vi "Start BaseActor.vi"() -> ()   [LabVIEW 2013, in "CS++Core-Examples.lvlib"]
doc: "This example illustrates how to start an actor via Factory and to send an Stop-Message on stop."
uses:
  CS++Core-Examples.lvlib
  Core/Classes/CS++BaseClasses/Factory/CS++Factory.lvclass
  Core/Classes/CS++BaseClasses/Factory/CS++Factory.lvclass/CS++Factory.ctl
  <vilib>/ActorFramework/Message Queue/Message Queue.lvclass/Message Queue.ctl
  <vilib>/ActorFramework/Message Enqueuer/Message Enqueuer.lvclass/Message Enqueuer.ctl
  <vilib>/ActorFramework/Message Enqueuer/Enqueue.vi
  <vilib>/Utility/config.llb/Read Key (String).vi
  <vilib>/ActorFramework/Message Priority Queue/Priority Enqueue.vi
  <vilib>/ActorFramework/Stop Msg/Stop Msg.lvclass
  <vilib>/ActorFramework/Actor/Actor.lvclass
  <vilib>/ActorFramework/Message Queue/Message Queue.lvclass
  Core/Libraries/MessageLogger/CS++MessageLogger.lvlib
  <vilib>/Utility/config.llb/NI_LVConfig.lvlib
panel:
  in  "Configuration File":path=path "C:/User/Brand/Git/CSPP/Core/CS++Example.ini"
  in  "Stop Button":bool
  in  "Object Name":string="myActor_0"
  out "Attributes found?":bool
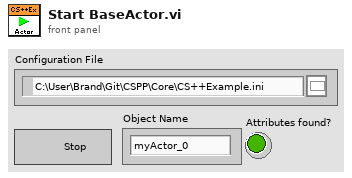
[diagram p1: front panel]
types:
  T1 = typedef "NI_LVConfig.lvlib/Config Data RefNum.ctl" = refnum<k1>
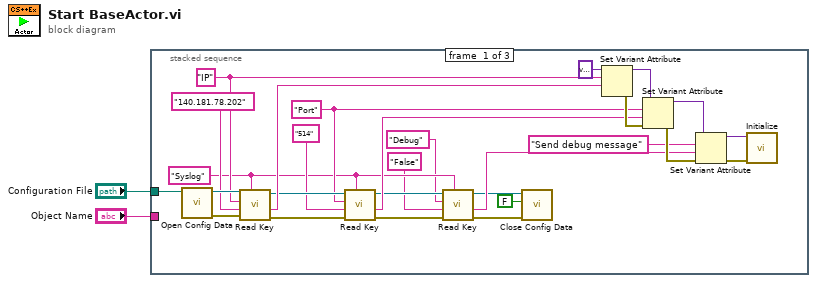
[diagram p0: block diagram]
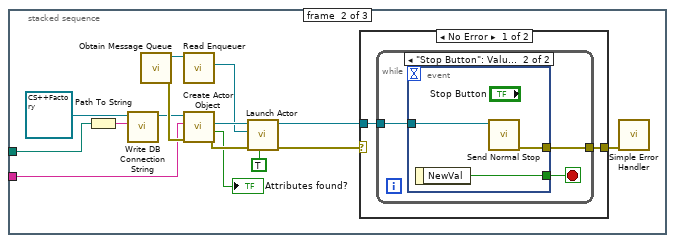
[diagram p2: hidden frame]
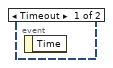
[diagram p3: hidden frame]
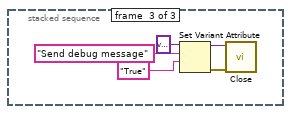
[diagram p5: hidden frame]
diagram:
  n1 = stacked-sequence {
    tunnel: "Object Name" -> [_ w39 _]
    tunnel: "Configuration File" -> [w22 w31 _]
    frame #0 {
      w9 = "Syslog" ("section")
      w14 = "Port" ("name")
      w19 = "IP" ("name")
      n2 = call <vilib>:"Open Config Data.vi"("configuration file path"=w22) -> ("error out"=w21:errorcluster, "refnum"=w20:T1)  [unwired: 8 in, 1 out]
      n3 = call-poly <vilib>:"Read Key.vi"("section"=w9, "error in (no error)"=w21, "default value"="140.181.78.202" ("name"), "key"=w19, "refnum"=w20) -> ("error out"=w15:errorcluster, "value"=w17:string, "refnum out"=w16:T1)  [unwired: 3 in, 1 out]
      n4 = call-poly <vilib>:"Read Key.vi"("section"=w9, "error in (no error)"=w15, "default value"="514" ("name"), "key"=w14, "refnum"=w16) -> ("error out"=w10:errorcluster, "value"=w12:string, "refnum out"=w11:T1)  [unwired: 3 in, 1 out]
      n5 = call-poly <vilib>:"Read Key.vi"("section"=w9, "error in (no error)"=w10, "default value"="False" ("name"), "key"="Debug", "refnum"=w11) -> ("error out"=w4:errorcluster, "value"=w6:string, "refnum out"=w5:T1)  [unwired: 3 in, 1 out]
      n6 = call <vilib>:"Close Config Data.vi"("error in (no error)"=w4, "write file if changed (T)"=FALSE, "refnum"=w5) -> ()  [unwired: 7 in, 2 out]
      n7 = Set Variant Attribute(Variant=variant ("variant"), name=w19, value=w17) -> (Variant out=w30:variant, error out=w29:errorcluster)  [unwired: 1 in, 1 out]
      n8 = Set Variant Attribute(Variant=w30, name=w14, value=w12, error in=w29) -> (Variant out=w28:variant, error out=w27:errorcluster)  [unwired: 1 out]
      n9 = Set Variant Attribute(Variant=w28, name="Send debug message", value=w6, error in=w27) -> (Variant out=w24:variant, error out=w23:errorcluster)  [unwired: 1 out]
      n10 = call "Initialize.vi"("Error In"=w23, "Initialization Data"=w24) -> ()  [unwired: 9 in, 1 out]
    }
    frame #1 {
      n11 = Path To String(path=w31) -> (string=w32:string)
      n12 = call "Write DB Connection String.vi"("DB Connection String"=w32, "CS++Factory in"=refnum<class "CS++Factory.lvclass"> refnum ("CS++BaseClasses.lvlib:CS++Factory.lvclass")) -> ("CS++Factory out"=w33:refnum<class "CS++Factory.lvclass">)  [unwired: 8 in, 1 out]
      n13 = call <vilib>:"Obtain Message Queue.vi"() -> ("error out"=w44:errorcluster, "Message Queue"=w45:refnum<class "Message Queue.lvclass">)  [unwired: 10 in]
      n14 = call <vilib>:"Read Enqueuer.vi"("Message Queue"=w45) -> ("Message Enqueuer"=w42:refnum<class "Message Enqueuer.lvclass">)  [unwired: 10 in]
      n15 = call "Create Actor Object.vi"("error in (no error)"=w44, "Object Name"=w39, "CS++Factory in"=w33) -> ("error out"=w41:errorcluster, "Attributes found?"=→"Attributes found?":bool, "C++BaseActor"=w43:refnum<class "CS++BaseActor.lvclass">)  [unwired: 5 in, 1 out]
      n16 = call <vilib>:"Launch Actor.vi"("Open Actor Core front panel? (F)"=TRUE, "error in (no error)"=w41, "Actor-to-Caller Enqueuer"=w42, "Actor"=w43) -> ("error out"=w37:errorcluster, "Caller-To-Actor Enqueuer"=w38:refnum<class "Message Enqueuer.lvclass">)  [unwired: 6 in]
      n17 = case shown="No Error" w37 {
        selector: w37 -> [_ w54]
        tunnel: w38 -> [w47 _]
        tunnel: [w46 w54] -> w36
        frame No Error {
          n18 = while {
            tunnel: w47 -> [w49]
            tunnel: [w48] -> w46
            stop <- w50 stop-if-true
            n19 = event shown="[1] \"Stop Button\": Value Change" {
              selector: _ -> [_ _]
              dyn-events: _ -> [_ _]
              timeout: _ -> [_ _]
              tunnel: [_ w53] -> w50
              tunnel: w49 -> [_ w52]
              tunnel: [_ w51] -> w48
              event Timeout {
                n20 = event-data() -> ()  [unwired: 1 in, 1 out]
              }
              event "Stop Button": Value Change {
                n21 = event-data() -> ("NewVal"=w53:bool)  [unwired: 1 in]
                n22 = call <vilib>:"Send Normal Stop.vi"("Message Enqueuer"=w52) -> ("error out"=w51:errorcluster)  [unwired: 10 in]
              }
            }
          }
        }
        frame Error {
        }
      }
      n23 = call <vilib>:"Simple Error Handler.vi"("error in (no error)"=w36) -> ()  [unwired: 4 in, 5 out]
    }
    frame #2 {
      n24 = Set Variant Attribute(Variant=variant ("variant"), name="Send debug message", value="True" ("name")) -> (Variant out=w57:variant, error out=w58:errorcluster)  [unwired: 1 in, 1 out]
      n25 = call "Close.vi"("Error In"=w58, "Initialization Data"=w57) -> ()  [unwired: 9 in, 1 out]
    }
  }
